vi "SCTL.vi"() -> ()   [LabVIEW 2012]
uses:
  <vilib>/Platform/TimedLoop/XDataNode/timing_clust.ctl
  <vilib>/Platform/TimedLoop/XDataNode/nitl_modes.ctl
  <vilib>/Platform/TimedLoop/XDataNode/wakeup.ctl
  <vilib>/rvi/FXPMathLib/basic elements/FxpIntAccumulator/subVIs/nifxpmath_IntAccumulator_SimConfig.ctl
  <vilib>/rvi/FXPMathLib/FxpSinAndCos/subVIs/nifxpmath_SinAndCos_SimConfig.ctl
  <vilib>/rvi/Emulation/niFpgaSctlEmulationRegisterWithScheduler.vi
  <vilib>/rvi/FXPMathLib/basic elements/FxpIntAccumulator/simVIs/DllFxpIntAccumulator_sub.vi
  <vilib>/rvi/FXPMathLib/FxpSinAndCos/simVIs/DllFxpSinAndCosTemp_sub.vi
  <vilib>/rvi/Emulation/niFpgaSctlEmulationScheduler.vi
  <vilib>/Platform/TimedLoop/XDataNode/XDataNode.xnode
  <vilib>/rvi/FXPMathLib/basic elements/FxpIntAccumulator/XNode/nifxpmath_IntAccumulator.xnode
  <vilib>/rvi/FXPMathLib/FxpSinAndCos/XNode/nifxpmath_SinAndCos.xnode
  <vilib>/Platform/TimedLoop/XDataNode/XDNodeRunTimeDep.lvlib
panel:
  out "Numeric 3":fxp<+/-,32,2>
  out "Numeric 2":fxp<+/-,32,32>
  out "Test Output":fxp<+/-,48,18>
  out "Numeric":fxp<+/-,32,2>
  in  "Input":fxp<+/-,16,16>
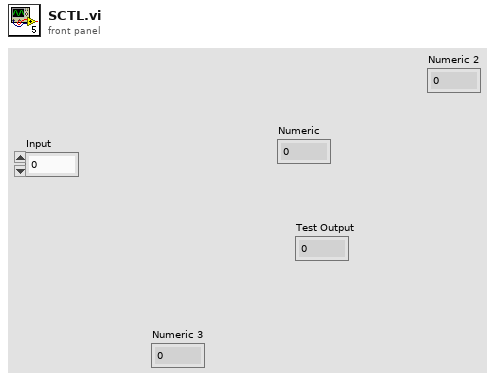
[diagram p1: front panel]
types:
  T1 = typedef "XDNodeRunTimeDep.lvlib/timing_clust.ctl" = cluster{"Expected End [f-1]":u64, "Actual End [f-1]":u64, "Finished Late? [f-1]":bool, "Expected End [i-1]":u64, "Actual End [i-1]":u64, "Finished Late? [i-1]":bool, "Expected Start [i]":u64, "Actual Start [i]":u64, "Expected Start [f]":u64, "Actual Start [f]":u64, "Source Name":string, "Structure Name":string, "Period":i64, "Deadline":i64, "Offset":i64, "Start":i64, "Priority":i32, "Timeout":i32, "Mode":T2, "Wakeup Reason":T3, "Error":errorcluster, "Source Type":string, "Secondary Source Type":string, "Global End Time":u64, "Global Start Time":u64, "Frame Duration":u64, "Iteration Duration":u64, "Assigned CPU":i32, "I/O Scan Engine Mode":u32}
  T2 = typedef "XDNodeRunTimeDep.lvlib/nitl_modes.ctl" = enum32{"No Change", "Process missed periods, maintain original phase", "Discard missed periods, maintain original phase", "Process missed periods, ignore original phase", "Discard missed periods, ignore original phase"}
  T3 = typedef "XDNodeRunTimeDep.lvlib/wakeup.ctl" = enum32{"Normal", "Aborted", "Asynchronous wakeup", "Timing source error", "Timed loop error", "Timeout"}
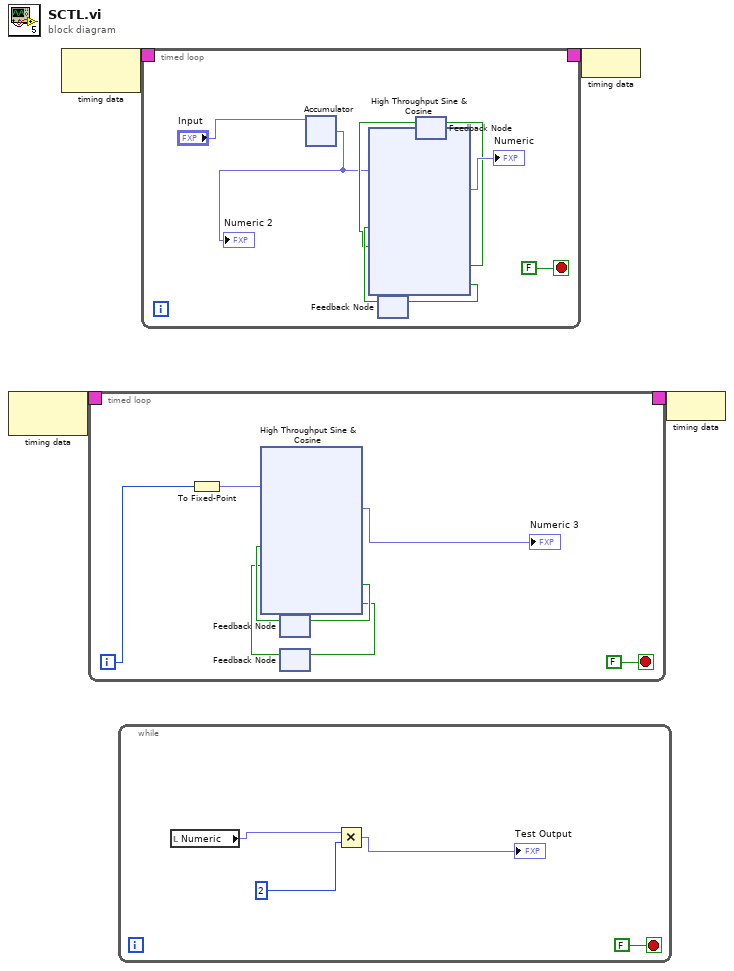
[diagram p0: block diagram]
diagram:
  n1 = node-c288() -> (w2:T1)  [unwired: 1 in]
  n2 = node-c288() -> (w4:T1)  [unwired: 1 in]
  n3 = timed-loop {
    timing: w2 -> [_]
    timing-out: [_] -> w1
    i -> [w5]
    stop <- FALSE stop-if-true
    n4 = To Fixed-Point(number=w5) -> (fixed-point=w6:fxp<+/-,32,32>)  [unwired: 1 in]
    n5 = feedback #1() -> (w11:bool)  [unwired: 1 in]
    n6 = feedback #2() -> (w9:bool)  [unwired: 1 in]
    n7 = xnode "High Throughput Sine & Cosine"("x (pi)"=w6, "input valid"=w11, "ready for output (T)"=w9) -> ("sin(x)"=→"Numeric 3":fxp<+/-,32,2>, "output valid"=w12:bool, "ready for input"=w10:bool)  [unwired: 1 out]
    n8 = feedback-in #1(w12) -> ()
    n9 = feedback-in #2(w10) -> ()
  }
  n10 = while {
    stop <- FALSE stop-if-true
    n11 = local read "Numeric"() -> (w49:fxp<+/-,32,2>)
    n12 = Multiply(x=w49, y=i16 2) -> (x*y=→"Test Output":fxp<+/-,48,18>)
  }
  n13 = timed-loop {
    timing: w4 -> [_]
    timing-out: [_] -> w3
    stop <- FALSE stop-if-true
    n14 = xnode "Accumulator"("x"="Input") -> ("s"=w51:fxp<+/-,32,32>)  [unwired: 4 in, 1 out]
    "Numeric 2" <- w51
    n15 = feedback #3() -> (w54:bool)  [unwired: 1 in]
    n16 = feedback #4() -> (w52:bool)  [unwired: 1 in]
    n17 = xnode ("High Throughput Sine & Cosine")("x (pi)"=w51, "input valid"=w54, "ready for output (T)"=w52) -> ("sin(x)"=→"Numeric":fxp<+/-,32,2>, "output valid"=w53:bool, "ready for input"=w55:bool)  [unwired: 1 out]
    n18 = feedback-in #3(w55) -> ()
    n19 = feedback-in #4(w53) -> ()
  }
  n20 = node-c288(w3) -> ()
  n21 = node-c288(w1) -> ()
